vi "Close Database.vi"(8 "error in (no error)":errorcluster, 11 ".NET Refnum in":refnum<k24>) -> (0 "error out":errorcluster)   [LabVIEW 2017, in "VIs to Interface LabVIEW and MySQL dotNET Connector.lvlib"]
doc: "Close the reference to the database."
uses:
  VIs to Interface LabVIEW and MySQL dotNET Connector.lvlib
  MySql.Data
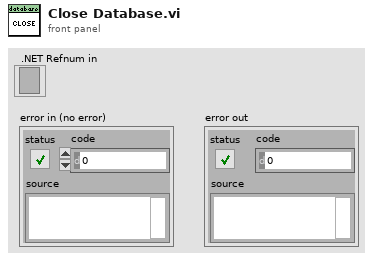
[diagram p1: front panel]
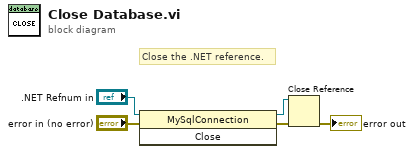
[diagram p0: block diagram]
diagram:
  # "Close the .NET reference."
  n1 = invoke class="MySqlConnection" method="Close"(reference=".NET Refnum in", error in="error in (no error)") -> (reference out=w4:refnum<k24>, error out=w3:errorcluster)  [unwired: 1 in, 1 out]
  n2 = Close Reference(reference=w4, error in (no error)=w3) -> (error out=→"error out":errorcluster)
